vi "Set Enable State on Multiple Controls.vi"(10 "启用？":bool, 11 "控件":refnum<vi>[](array[refnum])) -> ()   [LabVIEW 2020]
doc: "将输入数组中所有控件的值设置为“启用状态”。"
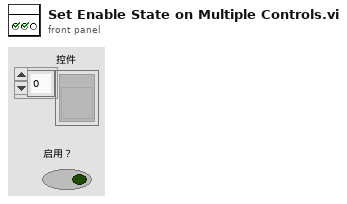
[diagram p1: front panel]
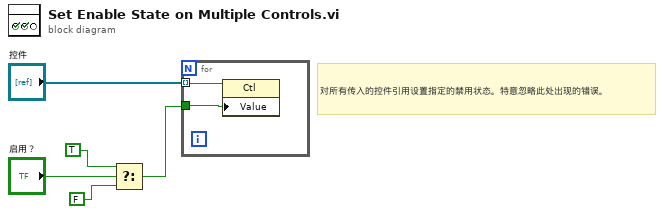
[diagram p0: block diagram]
diagram:
  # "对所有传入的控件引用设置指定的禁用状态。特意忽略此处出现的错误。"
  n1 = Select(t=TRUE, s="启用？", f=FALSE) -> (s? t:f=w3:bool)
  n2 = for {
    tunnel: "控件" -> [w7] mode=indexing
    tunnel: w3 -> [w6]
    n3 = property class="Ctl"(reference=w7, "Value"=w6) -> ()  [unwired: 1 in, 2 out]
  }
